vi "stageGoOrigin.vi"   [LabVIEW 2016]
uses:
  variables/applicationControl.vi
  variables/configDB.vi
  <vilib>/Instr/_visa.llb/VISA Configure Serial Port (Instr).vi
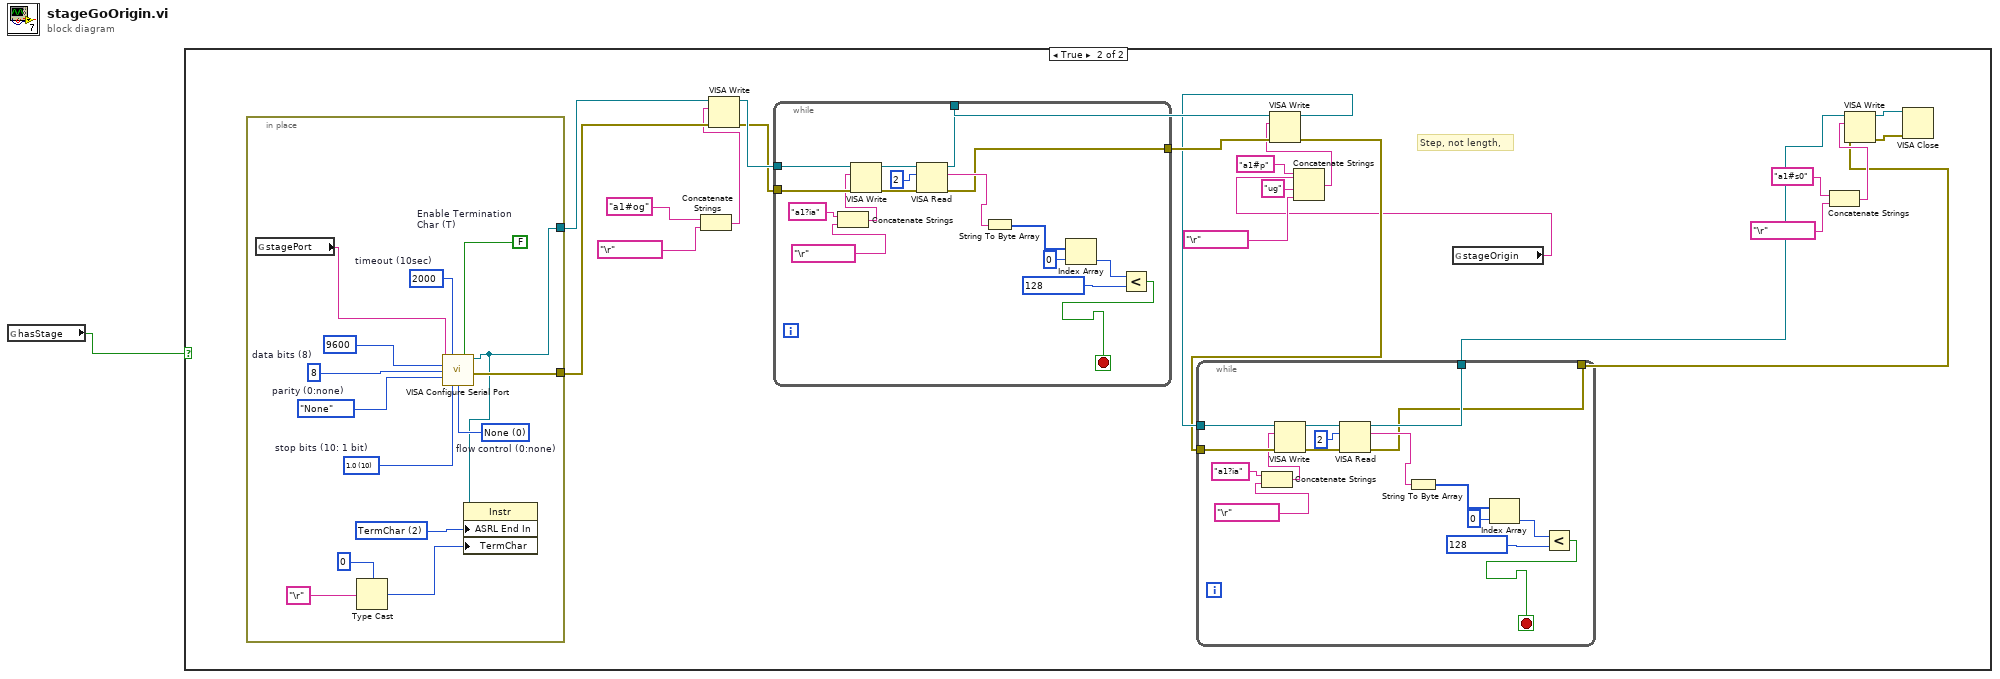
[diagram p0: block diagram]
diagram:
  n1 = global read "applicationControl.vi" "hasStage"() -> (w1:bool)
  n2 = case shown="True" w1 {
    frame False {
    }
    frame True {
      # "Step, not length,"
      n3 = in-place {
        in-place-border: [w58] -> w24
        in-place-border: [w63] -> w23
        w59 = u16 2 items=["None", "Last Bit", "TermChar"] ("Serial Settings:End Mode for Reads")
        w64 = u16 0 items=["None", "XON/XOFF", "RTS/CTS", "XON/XOFF & RTS/CTS", "DTR/DSR", "XON/XOFF & DTR/DSR"]  # flow control (0:none)
        w65 = u16 10 items=["1.0"=10, "1.5"=15, "2.0"=20]  # stop bits (10: 1 bit)
        w66 = FALSE  # Enable Termination Char (T)
        w67 = u32 2000  # timeout (10sec)
        w68 = enum16{"None", "Odd", "Even", "Mark", "Space"}."None"  # parity (0:none)
        w69 = u16 8  # data bits (8)
        n4 = global read "configDB.vi" "stagePort"() -> (w57:string)
        n5 = Type Cast(type=u8 0, x="\r") -> (*(type *) &x=w61:u8)
        n6 = call-poly "VISA Configure Serial Port"("VISA resource name"=w57, "timeout (10sec)"=w67, "Enable Termination\nChar (T)"=w66, "baud rate (9600)"=u32 9600, "data bits (8)"=w69, "parity (0:none)"=w68, "stop bits (10: 1 bit)"=w65, "flow control (0:none)"=w64) -> ("VISA resource name out"=w58:refnum<visa-resource-name>, "error out"=w63:errorcluster)  [unwired: 6 in]
        n7 = property class="Instr"(reference=w58, "ASRL End In"=w59, "TermChar"=w61) -> ()  [unwired: 1 in, 2 out]
      }
      n8 = Concatenate Strings("a1#og" ("string"), "\r" ("write buffer")) -> (w20:string)
      n9 = VISA Write(VISA resource name=w24, write buffer=w20, error in (no error)=w23) -> (VISA resource name out=w19:refnum<visa-resource-name>, error out=w18:errorcluster)  [unwired: 1 out]
      n10 = while {
        tunnel: w19 -> [w56]
        tunnel: w18 -> [w55]
        tunnel: [w48] -> w17
        tunnel: [w41] -> w16
        stop <- w42 stop-if-true
        n11 = Concatenate Strings("a1?ia" ("write buffer"), "\r" ("write buffer")) -> (w52:string)
        n12 = VISA Write(VISA resource name=w56, write buffer=w52, error in (no error)=w55) -> (VISA resource name out=w51:refnum<visa-resource-name>, error out=w50:errorcluster)  [unwired: 1 out]
        n13 = VISA Read(VISA resource name=w51, byte count=u32 2, error in (no error)=w50) -> (VISA resource name out=w48:refnum<visa-resource-name>, read buffer=w47:string, error out=w41:errorcluster)  [unwired: 1 out]
        n14 = String To Byte Array(string=w47) -> (unsigned byte array=w46:u8[])
        n15 = Index Array(array=w46, index=0) -> (element=w44:u8)
        n16 = Less?(x=w44, y=u8 128) -> (x < y?=w42:bool)
      }
      n17 = global read "configDB.vi" "stageOrigin"() -> (w2:string)
      n18 = Concatenate Strings("a1#p" ("string"), w2, "ug" ("string"), "\r" ("write buffer")) -> (w12:string)
      n19 = VISA Write(VISA resource name=w17, write buffer=w12, error in (no error)=w16) -> (VISA resource name out=w6:refnum<visa-resource-name>, error out=w5:errorcluster)  [unwired: 1 out]
      n20 = while {
        tunnel: w6 -> [w40]
        tunnel: w5 -> [w39]
        tunnel: [w32] -> w4
        tunnel: [w25] -> w3
        stop <- w26 stop-if-true
        n21 = Concatenate Strings("a1?ia" ("write buffer"), "\r" ("write buffer")) -> (w36:string)
        n22 = VISA Write(VISA resource name=w40, write buffer=w36, error in (no error)=w39) -> (VISA resource name out=w35:refnum<visa-resource-name>, error out=w34:errorcluster)  [unwired: 1 out]
        n23 = VISA Read(VISA resource name=w35, byte count=u32 2, error in (no error)=w34) -> (VISA resource name out=w32:refnum<visa-resource-name>, read buffer=w31:string, error out=w25:errorcluster)  [unwired: 1 out]
        n24 = String To Byte Array(string=w31) -> (unsigned byte array=w30:u8[])
        n25 = Index Array(array=w30, index=0) -> (element=w28:u8)
        n26 = Less?(x=w28, y=u8 128) -> (x < y?=w26:bool)
      }
      n27 = Concatenate Strings("a1#s0", "\r" ("write buffer")) -> (w7:string)
      n28 = VISA Write(VISA resource name=w4, write buffer=w7, error in (no error)=w3) -> (VISA resource name out=w11:refnum<visa-resource-name>, error out=w10:errorcluster)  [unwired: 1 out]
      n29 = VISA Close(VISA resource name=w11, error in (no error)=w10) -> ()  [unwired: 1 out]
    }
  }
